vi "Inv_Mpemba1_flat potential.vi"() -> ()   [LabVIEW 2019]
uses:
  <vilib>/eio/EIONode/EIONode.xnode
  <vilib>/rvi/eio/common/nirviEmuTemplateMethod_errors.vi
  <vilib>/eio/EIOPropertyNode/EIOPropertyNode.xnode
  <vilib>/rvi/eio/common/nirviEmuTemplatePropertyGet_errors.vi
  <vilib>/rvi/eio/common/nirviEmuTemplatePropertyGet_noerrors.vi
  <vilib>/rvi/eio/common/nirviEmuTemplatePropertySet_errors.vi
  <vilib>/rvi/eio/common/nirviEmuTemplatePropertySet_noerrors.vi
  <vilib>/rvi/DataTransferAndStorage/Container/XNode/niFpgaContainer.xnode
  <vilib>/rvi/FIFO/Fifo_Resource/nirvififoEmulationWrite.vi
  <vilib>/rvi/FIFO/Fifo_Resource/nirvififoEmulationRead.vi
  <vilib>/rvi/interface/RandomDataEmulation/nirviRandomDataFpgaReadWriteTemplate.vi
panel:
  in  "Xmin":sgl=-1.0
  in  "Fmax":sgl
  out "Fx out":sgl
  in  "Xmax":sgl=50.0
  in  "Enum":enum8{"No FB", "FB"}(ring)
  in  "MobX(px/V)":sgl
  in  "1/Xcali":sgl
  in  "Feedback parameters":T1
  in  "DX":sgl
  in  "DW":cluster{"xm":sgl, "Eb":sgl, "Tau":sgl, "dE":sgl}={"xm"=0.0, "Eb"=0.0, "Tau"=50.0, "dE"=0.0}
  in  "Xmean":sgl
  in  "Frequency":u32=100000
  in  "Triangle wave":T2={"signal offset_X"=5.0, "Scale X"=0.0, "signal offset_Y"=5.0, "Scale Y"=0.0, "Phase Shift"=30}
  in  "Xoffset":sgl
  in  "Yoffset":sgl
  in  "sum_offset":sgl
  in  "Normalize signal":bool=TRUE
  in  "FB Time":u8=5 caption="Feedback loop time"
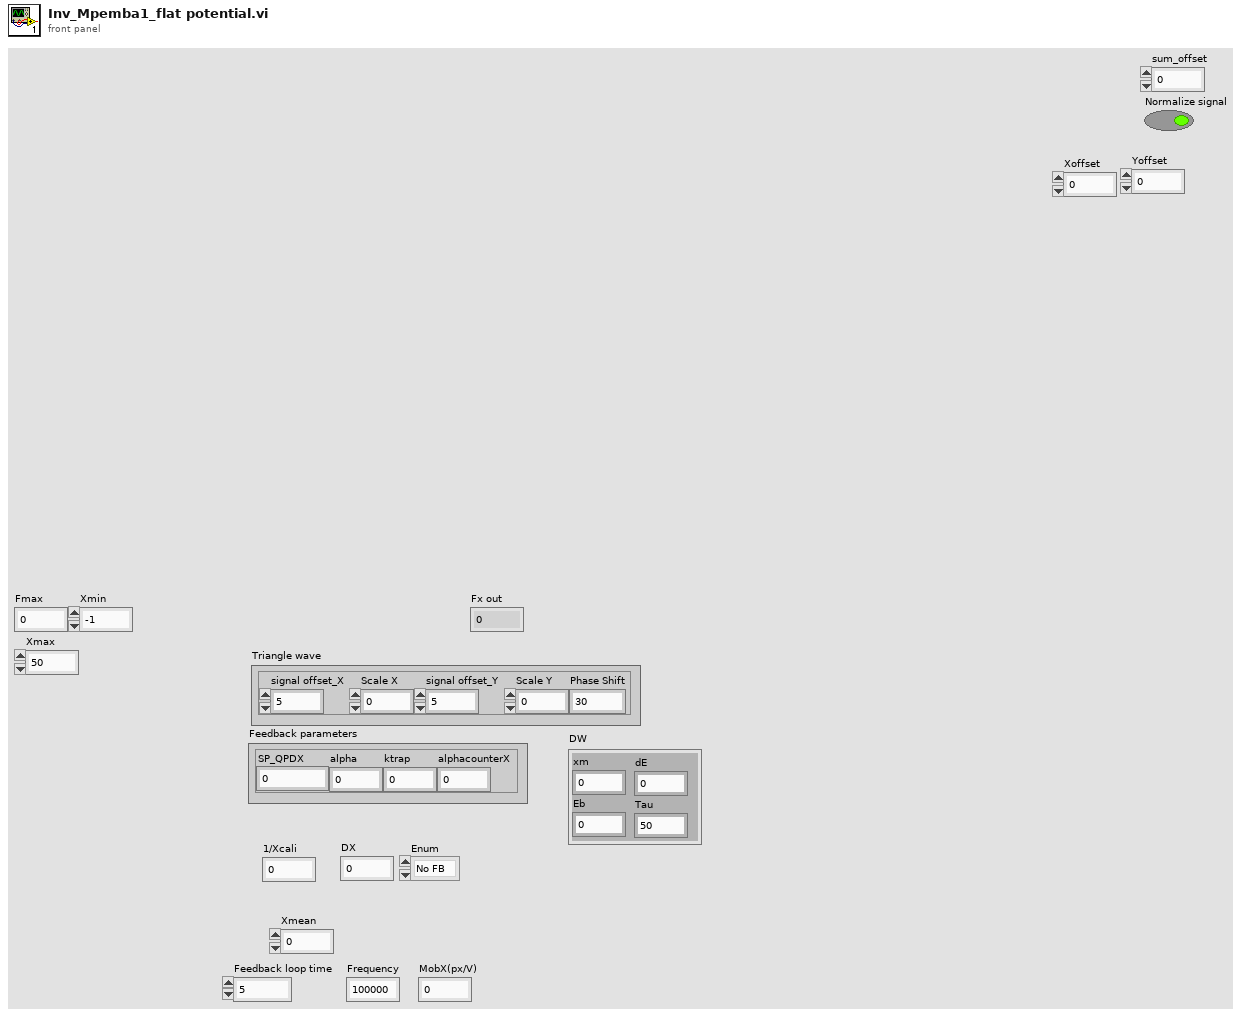
[diagram p1: front panel]
types:
  T1 = cluster{"SP_QPDX":sgl, "alpha":sgl, "ktrap":sgl, "alphacounterX":sgl}
  T2 = cluster{"signal offset_X":sgl, "Scale X":sgl, "signal offset_Y":sgl, "Scale Y":sgl, "Phase Shift":u32}
  T3 = enum8{"+/- 10 V", "+/- 5 V", "+/- 2 V", "+/- 1 V"}
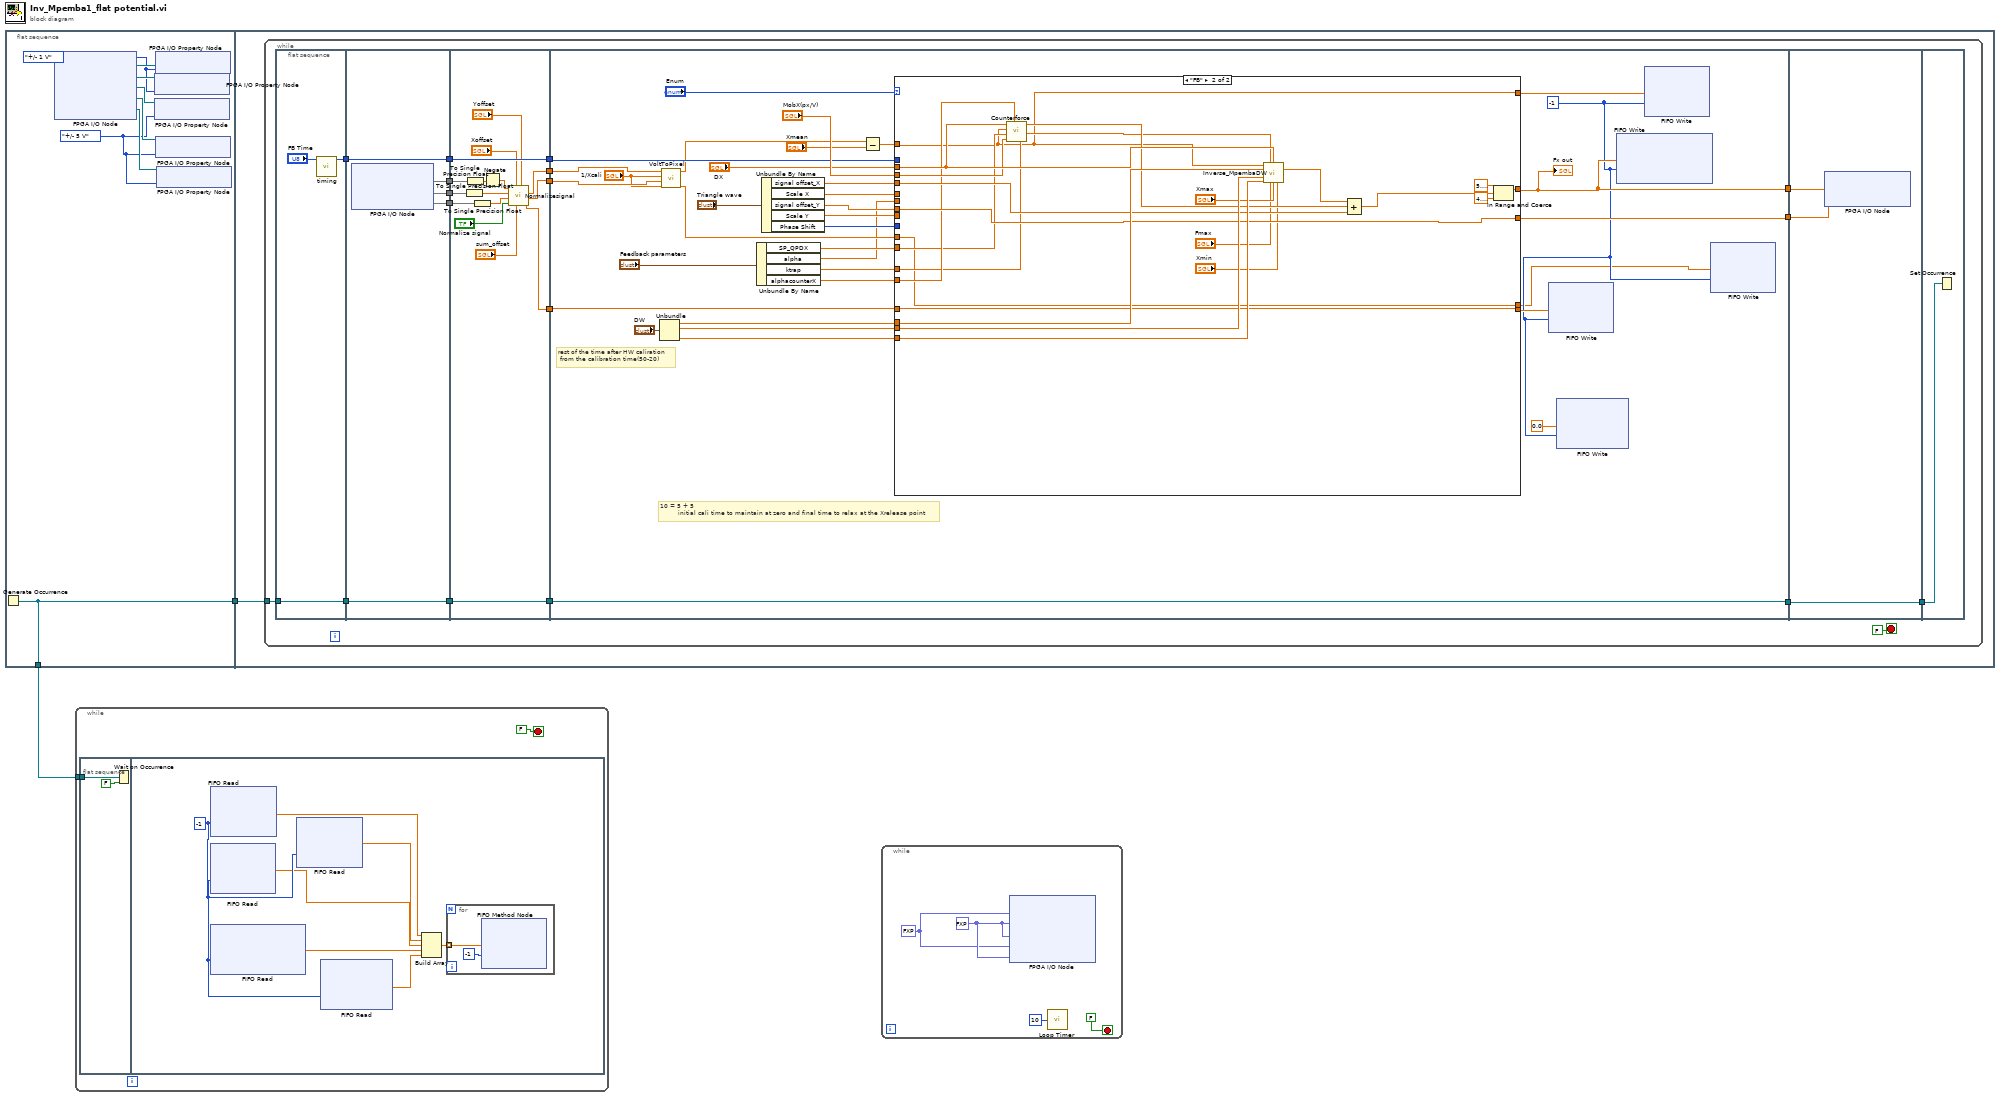
[diagram p0: block diagram]
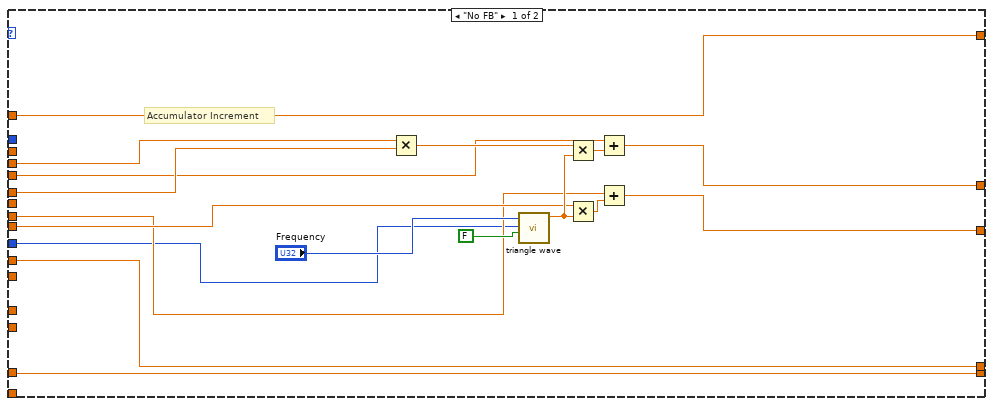
[diagram p2: hidden frame]
diagram:
  n1 = flat-sequence {
    tunnel: [w3] -> w1
    tunnel: [w3] -> w2
    tunnel: w1 -> [w11]
    frame #0 {
      w4 = T3."+/- 5 V" ("Voltage Range")
      w7 = T3."+/- 1 V" ("Voltage Range")
      n2 = Generate Occurrence() -> (w3:refnum<k4>)
      n3 = xnode "FPGA I/O Node"() -> ("FPGA I/O Out"=w10:refnum<k21>, "FPGA I/O Out"=w8:refnum<k21>, "FPGA I/O Out"=w9:refnum<k21>, "FPGA I/O Out"=w5:refnum<k21>, "FPGA I/O Out"=w6:refnum<k21>)  [unwired: 5 in, 5 out]
      n4 = xnode "FPGA I/O Property Node"("FPGA I/O In"=w8, "Voltage Range"=w7) -> ()  [unwired: 1 out]
      n5 = xnode "FPGA I/O Property Node"("FPGA I/O In"=w9, "Voltage Range"=w4) -> ()  [unwired: 1 out]
      n6 = xnode "FPGA I/O Property Node"("FPGA I/O In"=w10, "Voltage Range"=w7) -> ()  [unwired: 1 out]
      n7 = xnode "FPGA I/O Property Node"("FPGA I/O In"=w5, "Voltage Range"=w4) -> ()  [unwired: 1 out]
      n8 = xnode "FPGA I/O Property Node"("FPGA I/O In"=w6, "Voltage Range"=w4) -> ()  [unwired: 1 out]
    }
    frame #1 {
      n9 = while {
        tunnel: w11 -> [w17]
        stop <- FALSE ("stop") stop-if-true
        n10 = flat-sequence {
          tunnel: [w31] -> w18
          tunnel: w17 -> [w30]
          tunnel: [w30] -> w16
          tunnel: [w37] -> w28
          tunnel: [w36] -> w26
          tunnel: [w35] -> w24
          tunnel: [w34] -> w19
          tunnel: w18 -> [w34]
          tunnel: w16 -> [w33]
          tunnel: [w33] -> w15
          tunnel: w28 -> [w44]
          tunnel: [w52] -> w27
          tunnel: w26 -> [w43]
          tunnel: [w51] -> w25
          tunnel: w24 -> [w41]
          tunnel: [w50] -> w23
          tunnel: [w53] -> w20
          tunnel: w19 -> [w53]
          tunnel: w15 -> [w49]
          tunnel: [w49] -> w14
          tunnel: w27 -> [w84]
          tunnel: w25 -> [w83]
          tunnel: w23 -> [w80]
          tunnel: [w76] -> w22
          tunnel: [w88] -> w21
          tunnel: w20 -> [w85]
          tunnel: w14 -> [w73]
          tunnel: [w73] -> w12
          tunnel: w21 -> [w130]
          tunnel: w22 -> [w131]
          tunnel: [w129] -> w13
          tunnel: w12 -> [w129]
          tunnel: w13 -> [w132]
          frame #0 {
            n11 = call "timing.vi"("Feedback loop time"="FB Time") -> ("Feedback Loop time"=w31:u32)  [unwired: 10 in]
          }
          frame #1 {
            n12 = xnode "FPGA I/O Node"() -> ("Connector1/AI2"=w37, "Connector1/AI4"=w36, "Connector1/AI5"=w35)  [unwired: 3 in, 3 out]
          }
          frame #2 {
            n13 = To Single Precision Float(number=w43) -> (single precision float=w42:sgl)
            n14 = To Single Precision Float(number=w44) -> (single precision float=w39:sgl)
            n15 = To Single Precision Float(number=w41) -> (single precision float=w40:sgl)
            n16 = Negate(x=w39) -> (-x=w38:sgl)
            n17 = call "Normalizesignal.vi"("Yoffset"="Yoffset", "sum_offset"="sum_offset", "Xoffset"="Xoffset", "Normalize signal"="Normalize signal", "Sum"=w40, "Y"=w42, "X"=w38) -> ("Sum"=w50:sgl, "Y"=w51:sgl, "X"=w52:sgl)  [unwired: 2 in]
          }
          frame #3 {
            w67 = -1 ("Timeout")
            # "rest of the time after HW caliration\n from the calibration time(50-20)"
            # "10 = 5 + 5\n         initial cali time to maintain at zero and final time to relax at the Xrelease point"
            n18 = Unbundle("DW") -> ("xm"=w69:sgl, "Eb"=w81:sgl, "dE"=w74:sgl)  [unwired: 1 out]
            n19 = call "VoltToPixel.vi"("1/(QPDY/px)"="1/Xcali", "Normalized Y"=w83, "1/(QPDX/px)"="1/Xcali", "Normalized X"=w84) -> ("Ypx"=w82:sgl, "Xpx"=w71:sgl)  [unwired: 6 in]
            n20 = Unbundle By Name("Feedback parameters") -> ("SP_QPDX"=w59:sgl, "alpha"=w56:sgl, "ktrap"=w57:sgl, "alphacounterX"=w58:sgl)
            n21 = Unbundle By Name("Triangle wave") -> ("signal offset_X"=w63:sgl, "Scale X"=w65:sgl, "signal offset_Y"=w62:sgl, "Scale Y"=w64:sgl, "Phase Shift"=w61:u32)
            n22 = Subtract(x=w71, y="Xmean") -> (x-y=w78:sgl)
            n23 = case shown="\"FB\"" "Enum" {
              tunnel: w78 -> [w103 w107]
              tunnel: [w96 w121] -> w76
              tunnel: [w97 w119] -> w88
              tunnel: [w103 w107] -> w77
              tunnel: [w105 w111] -> w75
              tunnel: w80 -> [w105 w111]
              tunnel: w82 -> [w104 w112]
              tunnel: [w104 w112] -> w55
              tunnel: "MobX(px/V)" -> [w95 w126]
              tunnel: w85 -> [_ _]
              tunnel: "DX" -> [_ w127]
              tunnel: w69 -> [_ w124]
              tunnel: w81 -> [_ w128]
              tunnel: w74 -> [_ w125]
              tunnel: w65 -> [w93 _]
              tunnel: w64 -> [w92 _]
              tunnel: w63 -> [w91 w120]
              tunnel: w62 -> [w90 w119]
              tunnel: w61 -> [w89 _]
              tunnel: w59 -> [_ w113]
              tunnel: w58 -> [_ w118]
              tunnel: w57 -> [_ w117]
              tunnel: w56 -> [_ _]
              frame "No FB" {
                # "Accumulator Increment"
                n24 = Multiply(x=w95, y=w93) -> (x*y=w101:sgl)
                n25 = call "triangle wave.vi"("Reset Accumulator_TW"=FALSE, "phase shift"=w89, "Frequency"="Frequency") -> ("Tri wave out"=w98:sgl)  [unwired: 8 in]
                n26 = Multiply(x=w101, y=w98) -> (x*y=w100:sgl)
                n27 = Multiply(x=w92, y=w98) -> (x*y=w102:sgl)
                n28 = Add(x=w91, y=w100) -> (x+y=w96:sgl)
                n29 = Add(x=w90, y=w102) -> (x+y=w97:sgl)
              }
              frame "FB" {
                n30 = call "Counterforce.vi"("ktrap"=w117, "alphacounterX"=w118, "mobX(px/V)"=w126, "SP_X"=w113, "Xpx"=w107, "Dx"=w127) -> ("ktrap*mob"=w122:sgl, "counter Force"=w123:sgl)  [unwired: 3 in, 1 out]
                n31 = call "Inverse_MpembaDW.vi"("Xpos"=w107, "ktrap*mob"=w122, 2:w127, "Xm"=w124, "Eb"=w128, "dE"=w125, "Fmax"="Fmax", "Xmax"="Xmax", "Xmin"="Xmin") -> ("DWvolt"=w110:sgl)  [unwired: 6 in]
                n32 = Compound Arithmetic op=ADD(w110, w123, w120) -> (w116:sgl)
                n33 = In Range and Coerce(upper limit=sgl 5.1, x=w116, lower limit=sgl 4.9) -> (coerced(x)=w121:sgl)  [unwired: 1 out]
              }
            }
            "Fx out" <- w76
            n34 = xnode ("FIFO Write")("Element"=w75, "Timeout"=w67) -> ()  [unwired: 1 in, 2 out]
            n35 = xnode ("FIFO Write")("Element"=sgl 0.0 ("f"), "Timeout"=w67) -> ()  [unwired: 1 in, 2 out]
            n36 = xnode ("FIFO Write")("Element"=w76, "Timeout"=w67) -> ()  [unwired: 1 in, 2 out]
            n37 = xnode ("FIFO Write")("Element"=w77, "Timeout"=w67) -> ()  [unwired: 1 in, 2 out]
            n38 = xnode ("FIFO Write")("Element"=w55, "Timeout"=w67) -> ()  [unwired: 1 in, 2 out]
          }
          frame #4 {
            n39 = xnode "FPGA I/O Node"("Connector1/AO7"=w131, "Connector1/AO6"=w130) -> ()  [unwired: 2 in, 2 out]
          }
          frame #5 {
            n40 = Set Occurrence(w132) -> ()
          }
        }
      }
    }
  }
  n41 = while {
    tunnel: w2 -> [w133]
    stop <- FALSE stop-if-true
    n42 = flat-sequence {
      tunnel: w133 -> [w136]
      frame #0 {
        n43 = Wait on Occurrence(1:FALSE ("ignore previous (T)"), 2:w136) -> ()  [unwired: 1 in, 1 out]
      }
      frame #1 {
        w139 = -1 ("Timeout")
        n44 = xnode ("FIFO Read")("Timeout"=w139) -> ("Element"=w137:sgl)  [unwired: 1 in, 2 out]
        n45 = xnode ("FIFO Read")("Timeout"=w139) -> ("Element"=w140:sgl)  [unwired: 1 in, 2 out]
        n46 = xnode ("FIFO Read")("Timeout"=w139) -> ("Element"=w141:sgl)  [unwired: 1 in, 2 out]
        n47 = xnode ("FIFO Read")("Timeout"=w139) -> ("Element"=w138:sgl)  [unwired: 1 in, 2 out]
        n48 = xnode ("FIFO Read")("Timeout"=w139) -> ("Element"=w142:sgl)  [unwired: 1 in, 2 out]
        n49 = Build Array(w141, w138, w137, w140, w142) -> (w143:sgl[])
        n50 = for {
          tunnel: w143 -> [w145] mode=indexing
          n51 = xnode ("FIFO Method Node")("Element"=w145, "Timeout"=-1) -> ()  [unwired: 1 in, 2 out]
        }
      }
    }
  }
  n52 = while {
    stop <- FALSE stop-if-true
    w146 = fxp<+,8,3> 2.5 ("Connector1/AO2")
    w147 = fxp<+,8,3> 5.0 ("Connector1/AO2")
    n53 = xnode "FPGA I/O Node"("Connector1/AO0"=w146, "Connector1/AO2"=w147, "Connector1/AO3"=w147, "Connector1/AO4"=w146, "Connector1/AO5"=w147) -> ()  [unwired: 5 in, 5 out]
    n54 = call "Loop Timer"("Count(uSec)"=u8 10) -> ()  [unwired: 1 out]
  }
